vi "Measure_R.vi"(8 "errin":errorcluster, 11 "VISA in":refnum<visa-resource-name>) -> (0 "errout":errorcluster, 3 "Measurement":dbl)   [LabVIEW 2020]
uses:
  <vilib>/Instr/_visa.llb/VISA Open Access Mode.ctl
  <instrlib>/Agilent 3446X Series/Public/Data/Read (Single Point).vi
  <instrlib>/Agilent 3446X Series/Agilent 3446X Series.lvlib
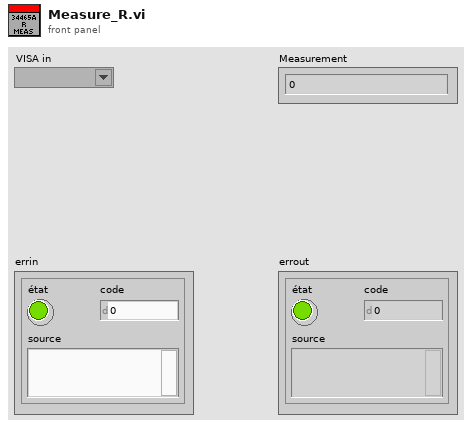
[diagram p1: front panel]
types:
  T1 = typedef "VISA Open Access Mode.ctl" = u32
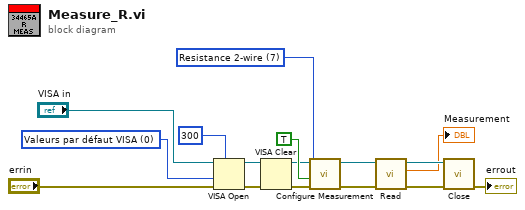
[diagram p0: block diagram]
diagram:
  w1 = 7 items=["Continuity", "Current AC", "Current DC", "Diode", "Frequency", "Resistance 4-wire", "Period", "Resistance 2-wire", "Temperature", "Voltage AC", "Voltage DC", "Voltage DC Ratio", "Capacitance"] ("Measurement Function (10: Voltage DC)")
  w6 = T1 0 items=["Valeurs par défaut VISA"=0, "Verrouillage exclusif"=1, "Charger les paramètres configurés"=4] ("Access Mode")
  n1 = VISA Open(timeout (0)=u32 300 ("Timeout de VISA Open (0)"), access mode=w6, error in (no error)="errin", VISA resource name="VISA in") -> (VISA resource name=w4:refnum<visa-resource-name>, error out=w5:errorcluster)  [unwired: 1 out]
  n2 = VISA Clear(VISA resource name=w4, error in (no error)=w5) -> (VISA resource name out=w9:refnum<visa-resource-name>, error out=w10:errorcluster)
  n3 = call <instrlib>:"Configure Measurement.vi"("error in (no error)"=w10, "Auto Range (T: Enable)"=TRUE, "Measurement Function (10: Voltage DC)"=w1, "VISA resource name"=w9) -> ("error out"=w11:errorcluster, "VISA resource name out"=w12:refnum<visa-resource-name>)  [unwired: 6 in]
  n4 = call-poly <instrlib>:"Read.vi"("error in (no error)"=w11, "VISA resource name"=w12) -> ("error out"=w14:errorcluster, "Measurement"=→"Measurement":dbl, "VISA resource name out"=w15:refnum<visa-resource-name>)  [unwired: 7 in]
  n5 = call <instrlib>:"Close.vi"("error in (no error)"=w14, "VISA resource name"=w15) -> ("error out"=→"errout":errorcluster)  [unwired: 9 in]
